vi "波形生成.vi"() -> ()   [LabVIEW 2011]
uses:
  <vilib>/measure/NI_MABase.lvlib
panel:
  in  "sampling info":cluster{"Fs":dbl, "#s":dbl}={"Fs"=1000.0, "#s"=1000.0} {"Fs" format="%.2p"}
  in  "stop":bool
  in  "phase":dbl format="%.2p"
  in  "amplitude":dbl=1.0 format="%0.2p"
  in  "frequency":dbl=10.0 format="%0.2p"
  in  "signal type":T1(ring)
  out "Waveform Chart":waveform(dbl)(graph)
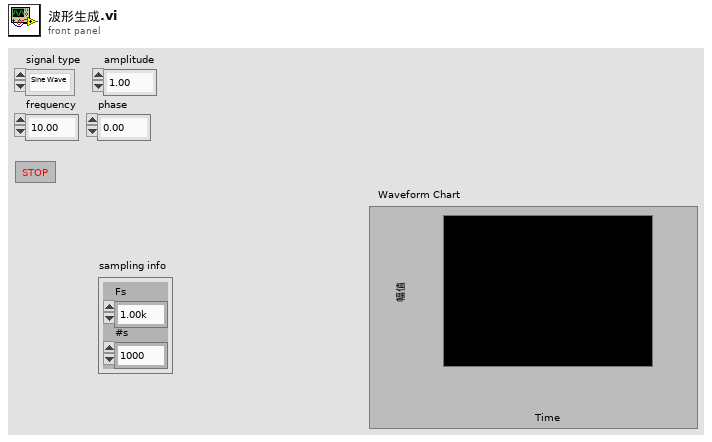
[diagram p1: front panel]
types:
  T1 = enum16{"Sine Wave", "Triangle Wave", "Square Wave", "Sawtooth Wave"}
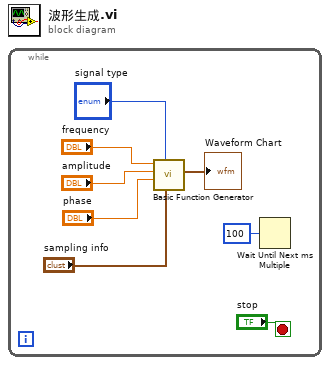
[diagram p0: block diagram]
diagram:
  n1 = while {
    stop <- "stop" stop-if-true
    n2 = call <vilib>:"Basic Function Generator.vi"("sampling info"="sampling info", "signal type"="signal type", "phase"="phase", "amplitude"="amplitude", "frequency"="frequency") -> ("signal out"=→"Waveform Chart":waveform(dbl))  [unwired: 4 in, 2 out]
    n3 = Wait Until Next ms Multiple(millisecond multiple=u32 100) -> ()  [unwired: 1 out]
  }
